vi "Prober_MoveToXYZTheta.vi"(6 "Theta location [mdeg]":string="none", 7 "SemiProbe in":refnum<class "SemiProbe.lvclass">, 8 "error in (no error)":errorcluster, 9 "Z location [µm]":string="none", 10 "Y location [µm]":string="none", 11 "X location [µm]":string="none") -> (0 "error out":errorcluster, 2 "String":string, 3 "SemiProbe out":refnum<class "SemiProbe.lvclass">)   [LabVIEW 2013, in "SemiProbe.lvclass"]
uses:
  SemiProbe.lvclass
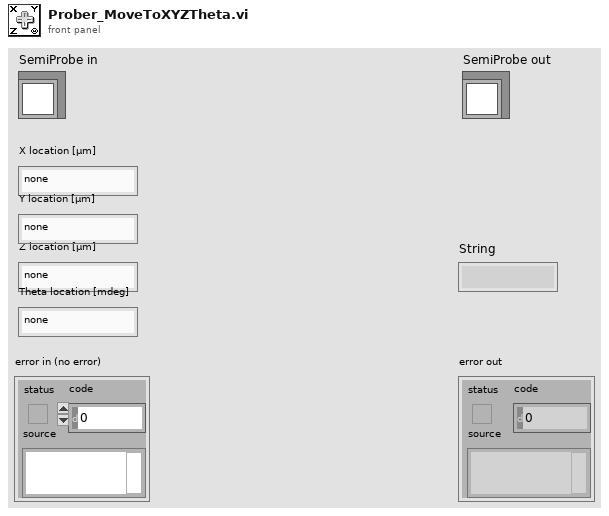
[diagram p1: front panel]
types:
  T1 = cluster{"SP Load Less Than Thr?":bool, "SP Load Threshold (um)":dbl, "SP Current Location":cluster{"X (um)":ext, "Y (um)":ext, "Z (um)":ext, "T (degree)":ext}, "SP Chuck Speeds":cluster{"XY Speed (10-100%)":dbl, "Z Speed (10-100%)":dbl, "T Speed (10-100%)":dbl}, "Manual Step Parameters":cluster{"Step in X":bool, "X S-Speed [µm/step]":sgl, "Step in Y":bool, "Y S-Speed [µm/step]":sgl, "Step in Z":bool, "Z S-Speed [µm/step]":sgl, "Step in T":bool, "T S-Speed [mdegree/step]":sgl, "X Increase":bool, "Y Increase?":bool, "Z Increase?":bool, "T Increase?":bool}, "Z Stepper":cluster{"UP/DOWN":bool, "UP/DOWN Speed [µm/step]":i32, "SP Z Step":bool}, "Z Heights Set":bool, "SP Contact Search":cluster{"Contact Circuit":enum16{"12", "1", "2"}, "Speed [1000-10000]":sgl, "Start Height [µm]":sgl, "Search Band [µm]":sgl, "Overdrive [µm]":sgl}, "Separation Distance [µm]":u32, "Contact Height [µm]":u32, "Use Overdrive?":bool, "Touchdown method":enum16{"no feedback", "Arduino edgesense", "SP contact circuit"}, "Arduino Edgesense params":cluster{"touchdown height [µm]":i32, "search band [µm]":u32, "speed [µm/step]":u32, "overdrive [µm]":u32}}
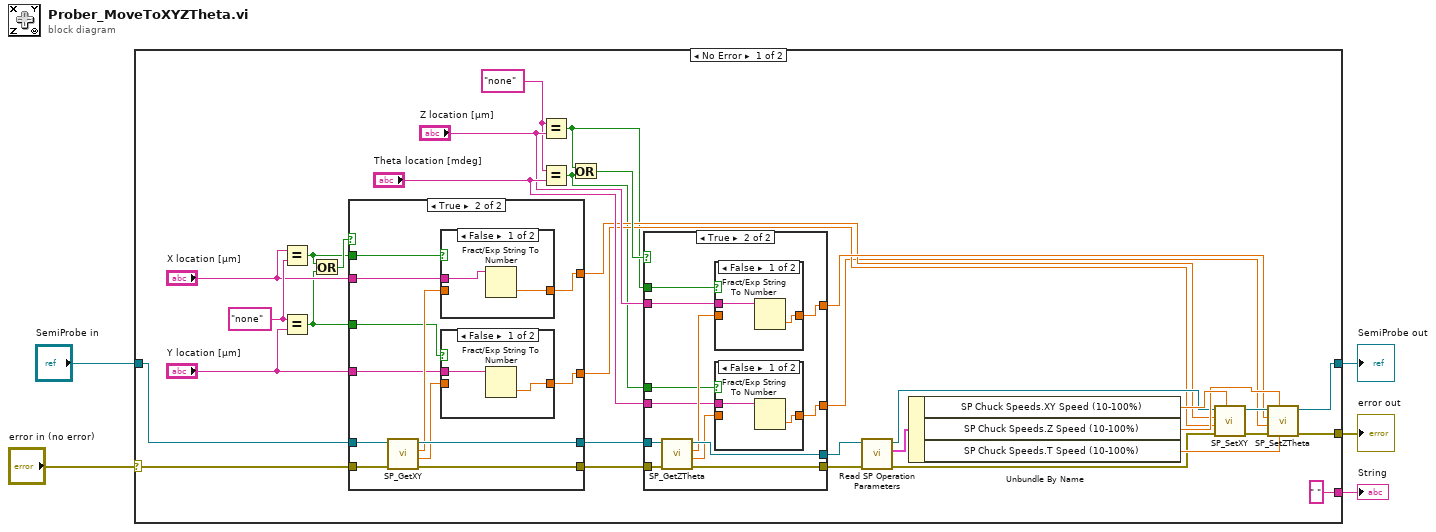
[diagram p0: block diagram]
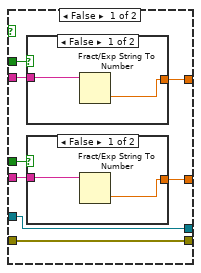
[diagram p2: hidden frame]
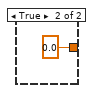
[diagram p3: hidden frame]
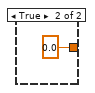
[diagram p4: hidden frame]
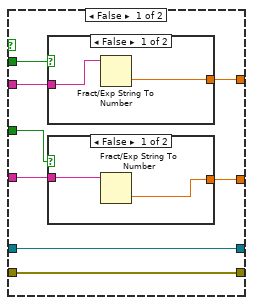
[diagram p7: hidden frame]
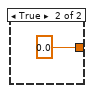
[diagram p8: hidden frame]
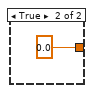
[diagram p9: hidden frame]
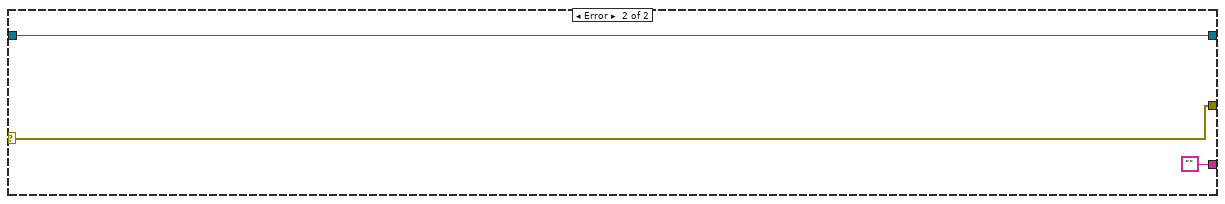
[diagram p12: hidden frame]
diagram:
  n1 = case shown="No Error" "error in (no error)" {
    selector: "error in (no error)" -> [w32 w105]
    tunnel: "SemiProbe in" -> [w31 w104]
    tunnel: [w21 w105] -> w3
    tunnel: [w20 w104] -> w2
    tunnel: [" " ""] -> w1
    frame No Error {
      w15 = "none"
      w23 = "none"
      n2 = Equal?(x="X location [µm]", y=w23) -> (x = y?=w10:bool)
      n3 = Equal?(x=w23, y="Y location [µm]") -> (x = y?=w9:bool)
      n4 = Or(x=w10, y=w9) -> (x .or. y?=w24:bool)
      n5 = case shown="True" w24 {
        tunnel: w32 -> [w76 w96]
        tunnel: w31 -> [w75 w95]
        tunnel: [w76 w94] -> w30
        tunnel: [w75 w93] -> w29
        tunnel: "X location [µm]" -> [w78 w90]
        tunnel: "Y location [µm]" -> [w77 w89]
        tunnel: [w74 w88] -> w12
        tunnel: [w73 w87] -> w13
        tunnel: w10 -> [w72 w86]
        tunnel: w9 -> [w71 w85]
        frame False {
          n6 = case shown="False" w72 {
            tunnel: w78 -> [w80 _]
            tunnel: [w79 0.0] -> w73
            frame False {
              n7 = Fract/Exp String To Number(string=w80) -> (number=w79:dbl)  [unwired: 3 in, 1 out]
            }
            frame True {
            }
          }
          n8 = case shown="False" w71 {
            tunnel: w77 -> [w83 _]
            tunnel: [w82 0.0] -> w74
            frame False {
              n9 = Fract/Exp String To Number(string=w83) -> (number=w82:dbl)  [unwired: 3 in, 1 out]
            }
            frame True {
            }
          }
        }
        frame True {
          n10 = call-dynamic "SP_GetXY.vi"("error in (no error)"=w96, "SemiProbe in"=w95) -> ("error out"=w94:errorcluster, "Y out"=w92:dbl, "X out"=w91:dbl, "SemiProbe out"=w93:refnum<class "SemiProbe.lvclass">)  [unwired: 6 in]
          n11 = case shown="False" w86 {
            tunnel: w91 -> [_ w102]
            tunnel: w90 -> [w101 _]
            tunnel: [w100 w102] -> w87
            frame False {
              n12 = Fract/Exp String To Number(string=w101) -> (number=w100:dbl)  [unwired: 3 in, 1 out]
            }
            frame True {
            }
          }
          n13 = case shown="False" w85 {
            tunnel: w92 -> [_ w99]
            tunnel: [w98 w99] -> w88
            tunnel: w89 -> [w97 _]
            frame False {
              n14 = Fract/Exp String To Number(string=w97) -> (number=w98:dbl)  [unwired: 3 in, 1 out]
            }
            frame True {
            }
          }
        }
      }
      n15 = Equal?(x=w15, y="Z location [µm]") -> (x = y?=w7:bool)
      n16 = Equal?(x=w15, y="Theta location [mdeg]") -> (x = y?=w8:bool)
      n17 = Or(x=w7, y=w8) -> (x .or. y?=w22:bool)
      n18 = case shown="True" w22 {
        tunnel: w30 -> [w45 w64]
        tunnel: w29 -> [w46 w63]
        tunnel: [w45 w62] -> w27
        tunnel: [w46 w61] -> w28
        tunnel: "Theta location [mdeg]" -> [w44 w58]
        tunnel: "Z location [µm]" -> [w42 w57]
        tunnel: [w43 w56] -> w6
        tunnel: [w41 w55] -> w14
        tunnel: w8 -> [w39 w54]
        tunnel: w7 -> [w40 w53]
        frame False {
          n19 = case shown="False" w40 {
            tunnel: w42 -> [w51 _]
            tunnel: [w50 0.0] -> w41
            frame False {
              n20 = Fract/Exp String To Number(string=w51) -> (number=w50:dbl)  [unwired: 3 in, 1 out]
            }
            frame True {
            }
          }
          n21 = case shown="False" w39 {
            tunnel: w44 -> [w48 _]
            tunnel: [w47 0.0] -> w43
            frame False {
              n22 = Fract/Exp String To Number(string=w48) -> (number=w47:dbl)  [unwired: 3 in, 1 out]
            }
            frame True {
            }
          }
        }
        frame True {
          n23 = call-dynamic "SP_GetZTheta.vi"("error in (no error)"=w64, "SemiProbe in"=w63) -> ("error out"=w62:errorcluster, "Theta out [mdeg]"=w59:dbl, "Z out [µm]"=w60:dbl, "SemiProbe out"=w61:refnum<class "SemiProbe.lvclass">)  [unwired: 6 in]
          n24 = case shown="False" w53 {
            tunnel: w60 -> [_ w70]
            tunnel: w57 -> [w69 _]
            tunnel: [w68 w70] -> w55
            frame False {
              n25 = Fract/Exp String To Number(string=w69) -> (number=w68:dbl)  [unwired: 3 in, 1 out]
            }
            frame True {
            }
          }
          n26 = case shown="False" w54 {
            tunnel: w59 -> [_ w67]
            tunnel: w58 -> [w66 _]
            tunnel: [w65 w67] -> w56
            frame False {
              n27 = Fract/Exp String To Number(string=w66) -> (number=w65:dbl)  [unwired: 3 in, 1 out]
            }
            frame True {
            }
          }
        }
      }
      n28 = call-dynamic "Read SP Operation Parameters.vi"("error in (no error)"=w27, "SemiProbe in"=w28) -> ("error out"=w25:errorcluster, "SP Operation Parameters"=w33:T1, "SemiProbe out"=w26:refnum<class "SemiProbe.lvclass">)  [unwired: 7 in]
      n29 = Unbundle By Name(w33) -> ("SP Chuck Speeds.XY Speed (10-100%)"=w38:dbl, "SP Chuck Speeds.Z Speed (10-100%)"=w34:dbl, "SP Chuck Speeds.T Speed (10-100%)"=w35:dbl)
      n30 = call-dynamic "SP_SetXY.vi"("XY Speed (10-100%)"=w38, "error in (no error)"=w25, "Y in um"=w12, "X in um"=w13, "SemiProbe in"=w26) -> ("error out"=w37:errorcluster, "SemiProbe out"=w36:refnum<class "SemiProbe.lvclass">)  [unwired: 5 in]
      n31 = call-dynamic "SP_SetZTheta.vi"("Theta Speed (10-100%)"=w35, "Z Speed (10-100%)"=w34, "error in (no error)"=w37, "Theta in mdeg"=w6, "Z in um"=w14, "SemiProbe in"=w36) -> ("error out"=w21:errorcluster, "SemiProbe out"=w20:refnum<class "SemiProbe.lvclass">)  [unwired: 4 in]
    }
    frame Error {
    }
  }
  "error out" <- w3
  "SemiProbe out" <- w2
  "String" <- w1
